vi "Write Current Section.vi"(8 "error in (no error)":errorcluster, 10 "Current Section":string, 11 "Config Data in":refnum<class "Config Data.lvclass">) -> (0 "error out":errorcluster, 3 "Config Data out":refnum<class "Config Data.lvclass">)   [LabVIEW 2014, in "Config Data.lvclass"]
uses:
  Config Data.lvclass
  Config Data.lvclass/Config Data.ctl
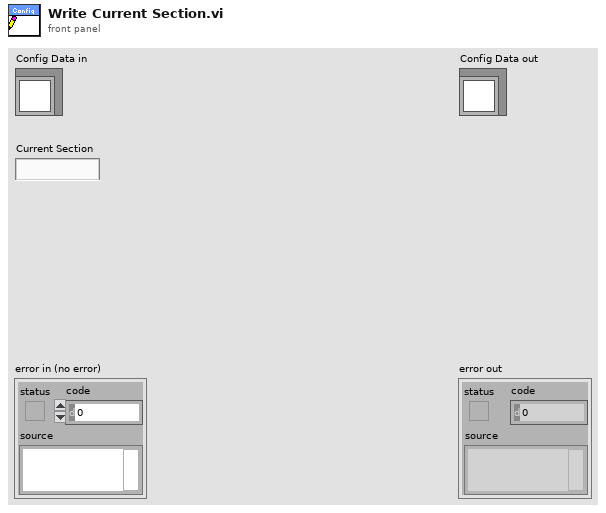
[diagram p1: front panel]
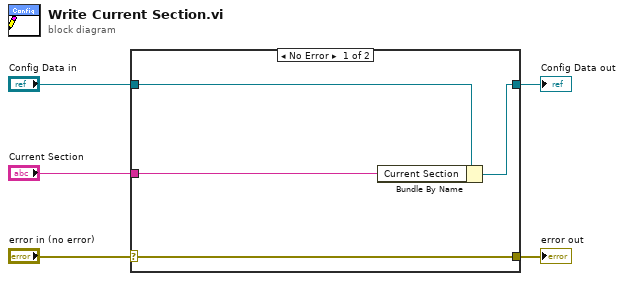
[diagram p0: block diagram]
diagram:
  n1 = case shown="No Error" "error in (no error)" {
    selector: "error in (no error)" -> [w9 w10]
    tunnel: [w9 w10] -> w4
    tunnel: [w7 w11] -> w2
    tunnel: "Config Data in" -> [w8 w11]
    tunnel: "Current Section" -> [w6 _]
    frame No Error {
      n2 = Bundle By Name(cluster=w8, "Current Section"=w6) -> (w7:refnum<class "Config Data.lvclass">)
    }
    frame Error {
    }
  }
  "error out" <- w4
  "Config Data out" <- w2
